vi "2B_Tech Serial Data Recording & DECADE 3.0.vi"() -> ()   [LabVIEW 2014]
uses:
  <vilib>/Instr/_visa.llb/VISA Set IO Buffer Mask.ctl
  <vilib>/Instr/_visa.llb/VISA Flush IO Buffer Mask.ctl
  <vilib>/Platform/TimedLoop/XDataNode/timing_clust.ctl
  <vilib>/Platform/TimedLoop/XDataNode/nitl_modes.ctl
  <vilib>/Platform/TimedLoop/XDataNode/wakeup.ctl
  C:/Program Files (x86)/National Instruments/LabVIEW 2014/examples/Data Communication/Network Streams/Simple Network Streams/support/Network Stream Command.ctl
  <vilib>/Utility/error.llb/whitespace.ctl
  <vilib>/Instr/_visa.llb/VISA Configure Serial Port (Instr).vi
  <vilib>/Utility/tcp.llb/UDP Multicast Write-Only Open.vi
  <vilib>/platform/TimedLoop/XDataNode/XDataNode.xnode
  <vilib>/Platform/TimedLoop/XDataNode/XDNodeRunTimeDep.lvlib
panel:
  out "SEPTIC TCP Error Out":errorcluster
  out "TCP packet\nSend to SEPTIC":bool
  in  "stop 2":bool
  out "FISH TCP Error Out":errorcluster
  out "TCP packet\nSend to FISH":bool
  in  "stop":bool
  out "Default file name":string
  out "error out":errorcluster
  out "Ambient/Cabin":bool
  out "Stop File Write":bool
  in  "timeout (10sec)":u32=3000
  in  "VISA resource name":refnum<visa-resource-name>="ASRL2::INSTR"
  out "Simulate 3 av":dbl
  out "Simulate\nConc":i32
  out "Simulate\nconc":bool
  out "3hr_alm_thresh":i32=80
  out "3hrAvg_Alarm":bool
  out "Inst_Alarm":bool
  out "Inst_alm_thresh":i32=220
  out "Time":string
  in  "Clear Display\nErrors":bool
  out "Read Error Counter\nfrom process loop":u32
  out "CABOZO UDP_ASCII_Out":string
  out "Ozo_array":string[](array[string])
  out "3hr_ozo_avg":dbl
  out "q_size":i32
  out "Data Output":string[](array[string])
  out "UDP packet\nSend status":bool
  out "TWBOZO UDP_ASCII_Out":string
  out "UDP_Out_Error":errorcluster
  out "UDP_Pack_num":u32
  out "Flight Number":string
  out "Number of times \nRead time out":u32
  out "Data Loop count":i32
  out "2B_Serial_error out":errorcluster
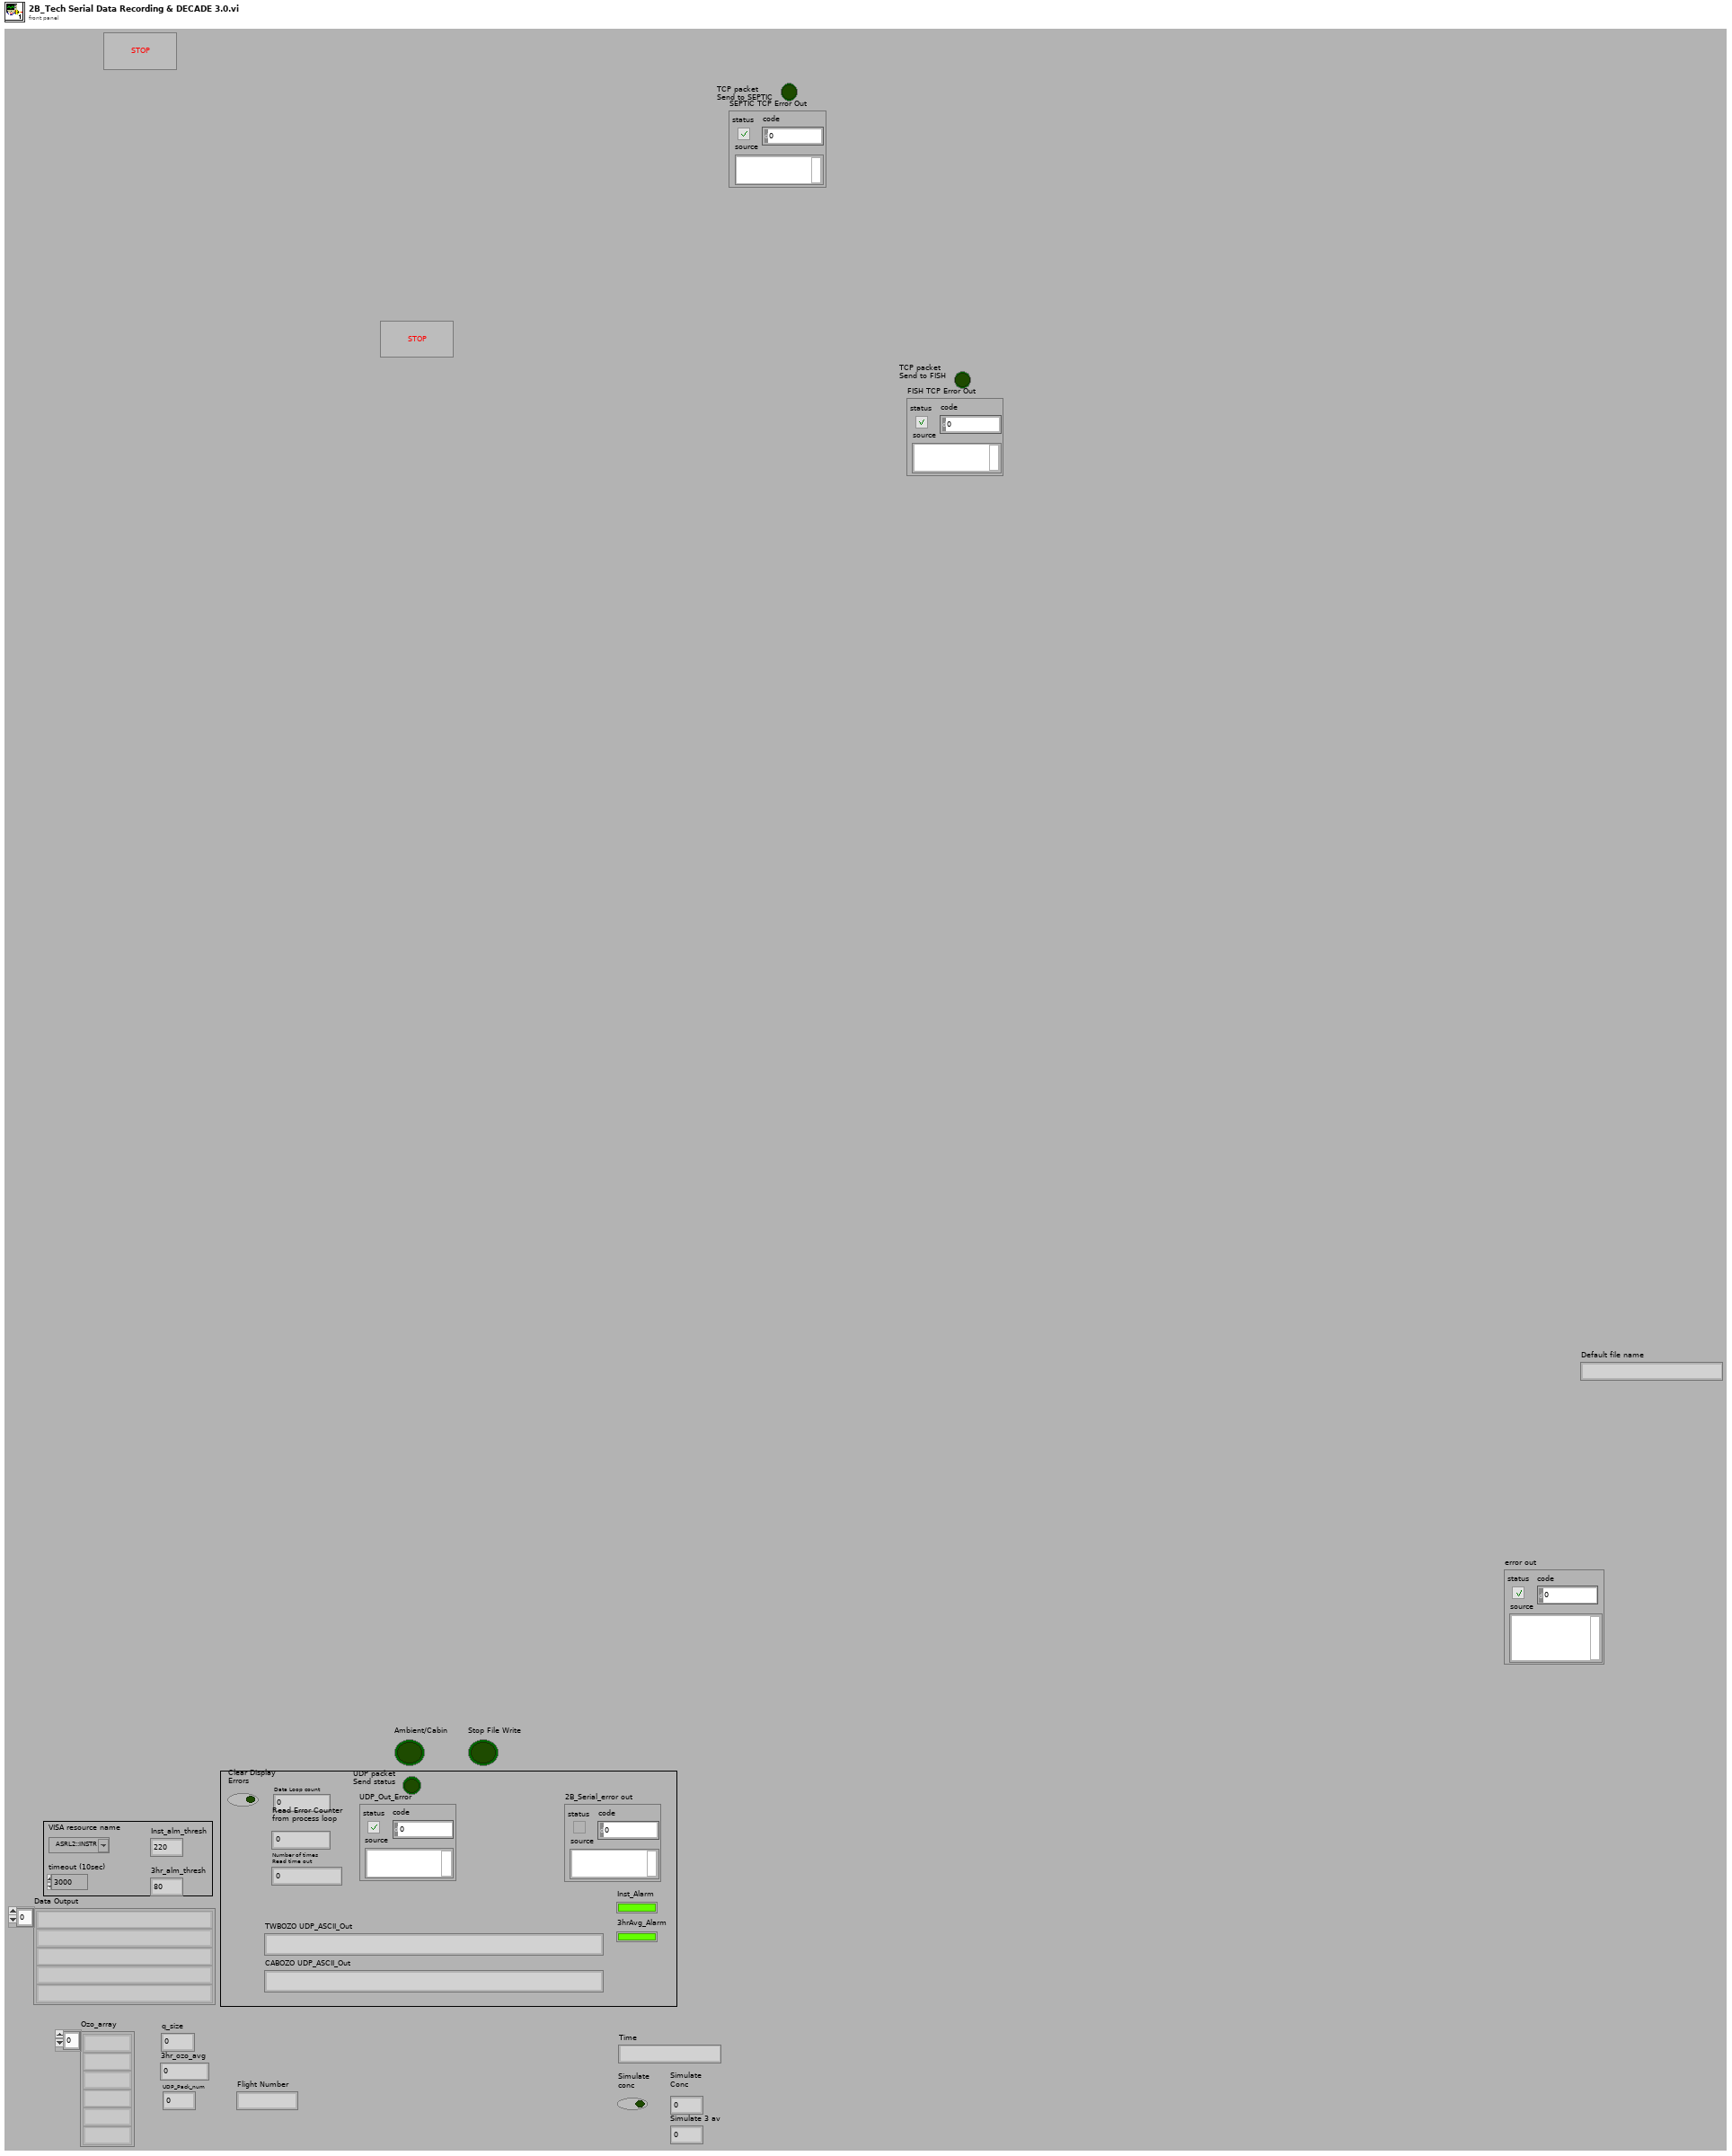
[diagram p1: front panel]
types:
  T1 = typedef "VISA Flush IO Buffer Mask.ctl" = u16
  T2 = typedef "VISA Set IO Buffer Mask.ctl" = u16
  T3 = typedef "XDNodeRunTimeDep.lvlib/timing_clust.ctl" = cluster{"Expected End [f-1]":u64, "Actual End [f-1]":u64, "Finished Late? [f-1]":bool, "Expected End [i-1]":u64, "Actual End [i-1]":u64, "Finished Late? [i-1]":bool, "Expected Start [i]":u64, "Actual Start [i]":u64, "Expected Start [f]":u64, "Actual Start [f]":u64, "Source Name":string, "Structure Name":string, "Period":i64, "Deadline":i64, "Offset":i64, "Start":i64, "Priority":i32, "Timeout":i32, "Mode":T4, "Wakeup Reason":T5, "Error":errorcluster, "Source Type":string, "Secondary Source Type":string, "Global End Time":u64, "Global Start Time":u64, "Frame Duration":u64, "Iteration Duration":u64, "Assigned CPU":i32, "I/O Scan Engine Mode":u32}
  T4 = typedef "XDNodeRunTimeDep.lvlib/nitl_modes.ctl" = enum32{"No Change", "Process missed periods, maintain original phase", "Discard missed periods, maintain original phase", "Process missed periods, ignore original phase", "Discard missed periods, ignore original phase"}
  T5 = typedef "XDNodeRunTimeDep.lvlib/wakeup.ctl" = enum32{"Normal", "Aborted", "Asynchronous wakeup", "Timing source error", "Timed loop error", "Timeout"}
  T6 = typedef "Network Stream Command.ctl" = cluster{"Message":string, "Message Data":variant}
  T7 = enum16{"open", "replace", "create", "open or create", "replace or create", "replace or create with confirmation"}
  T8 = typedef "whitespace.ctl" = u16
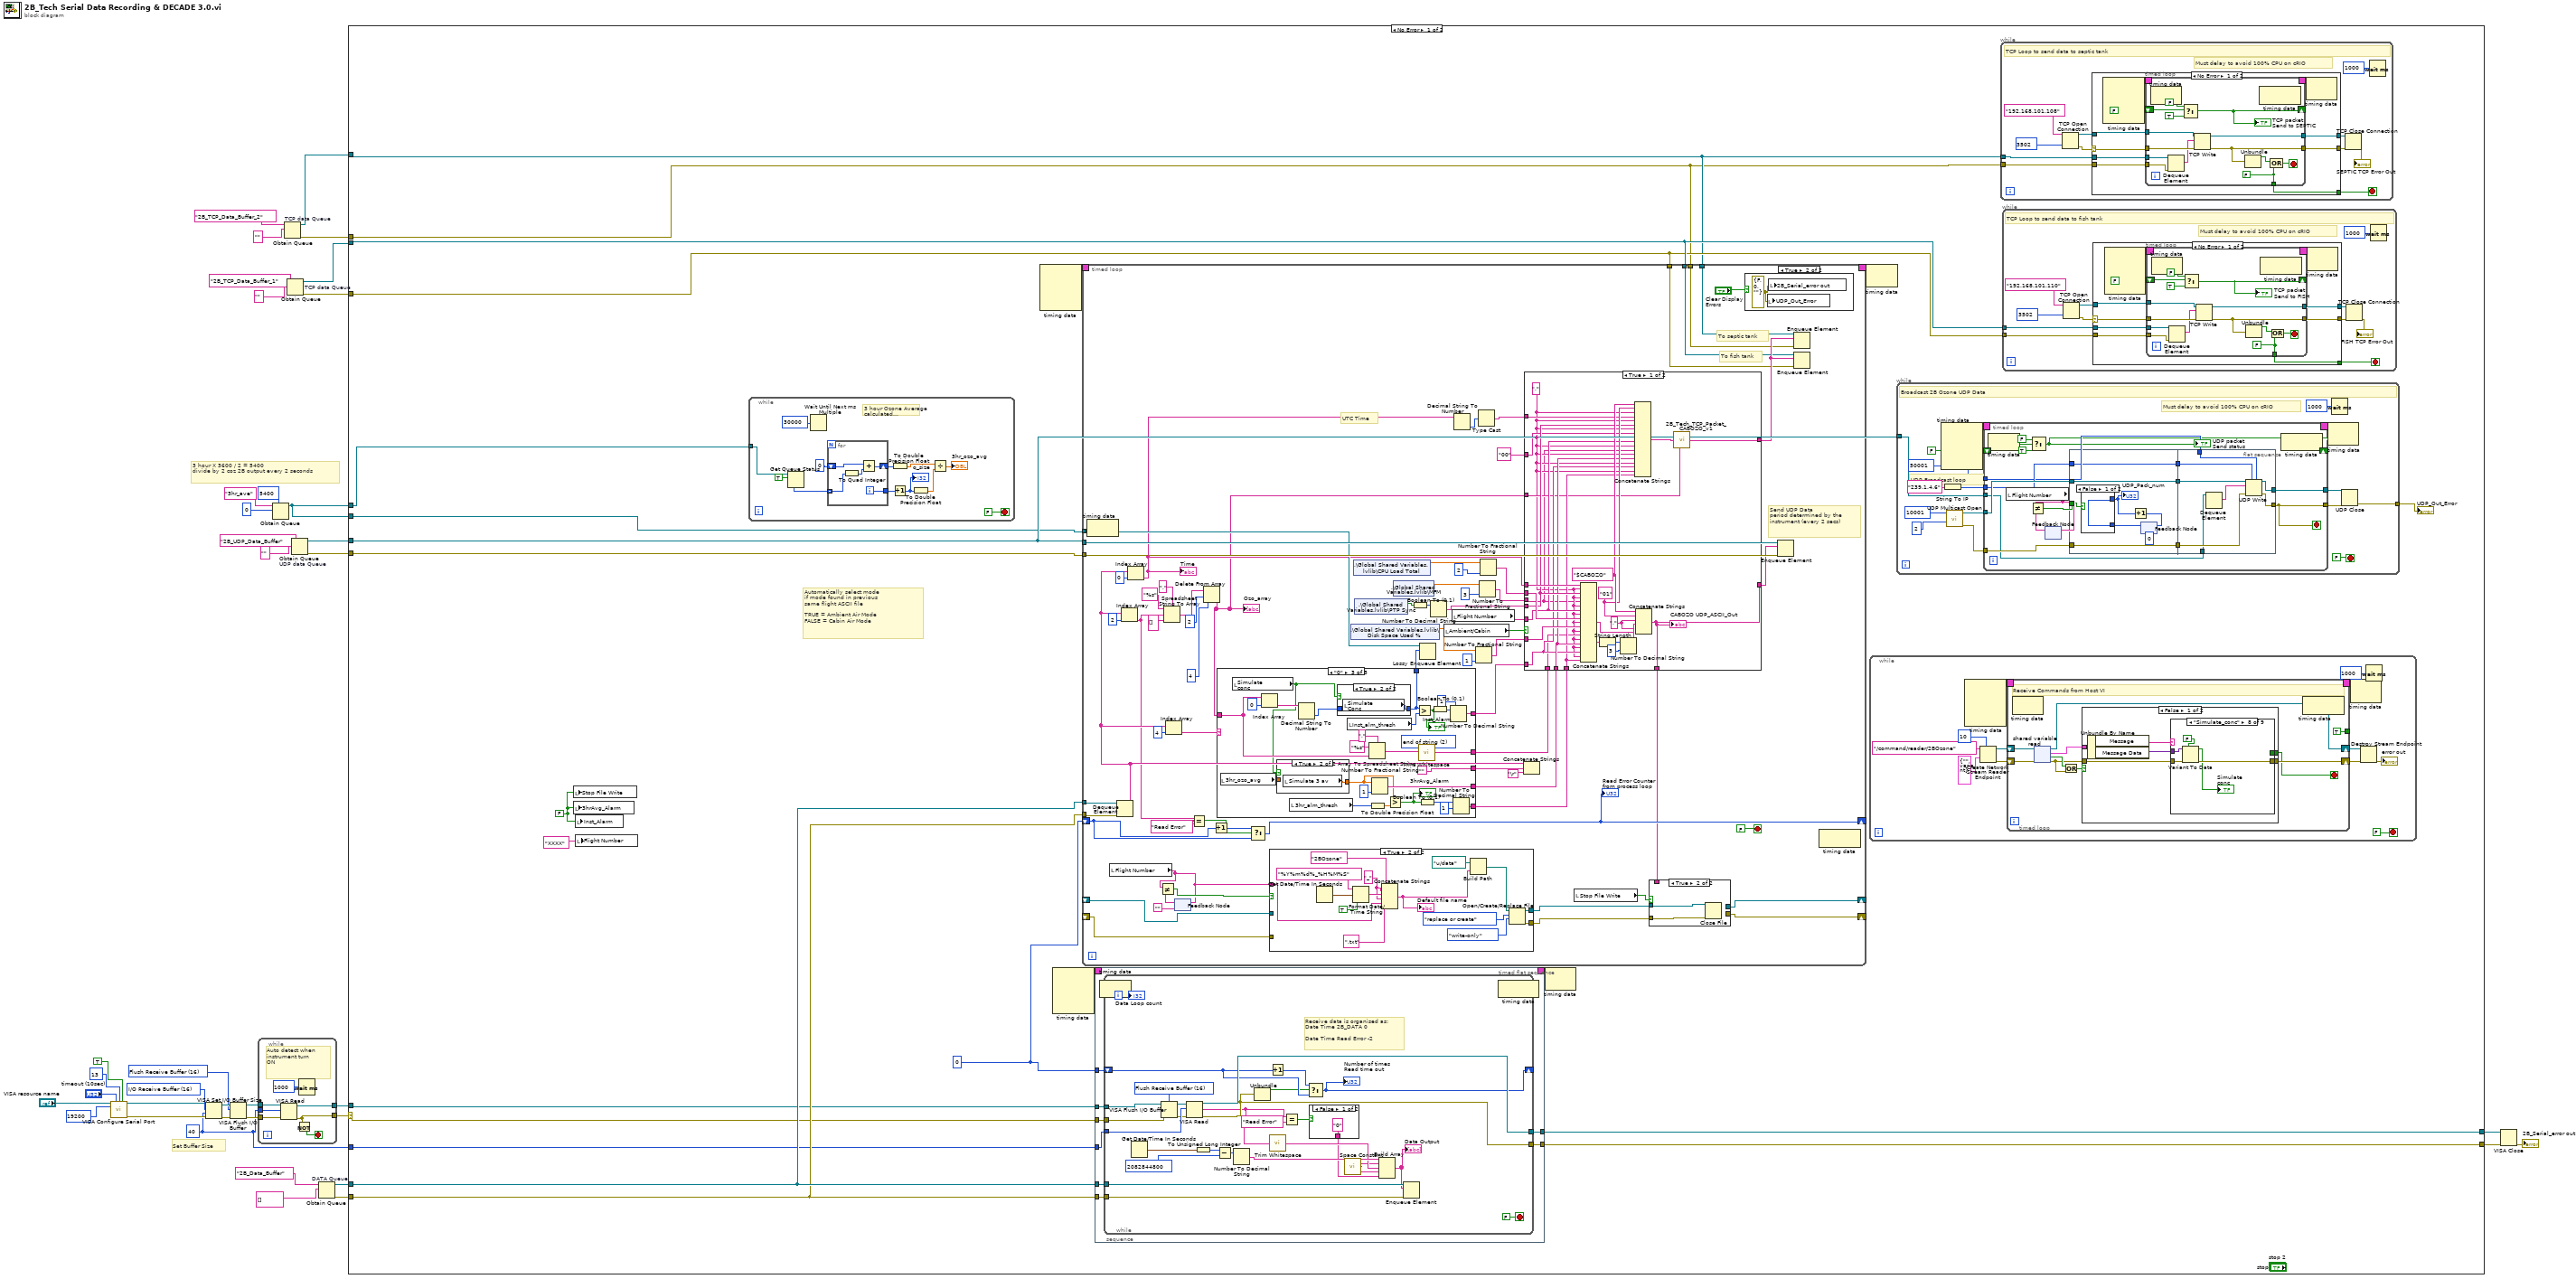
[diagram p0: block diagram]
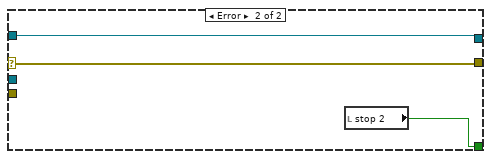
[diagram p2: hidden frame]
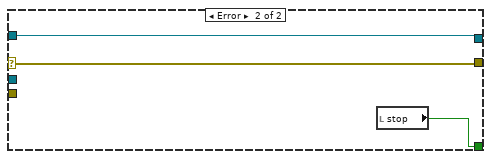
[diagram p3: hidden frame]
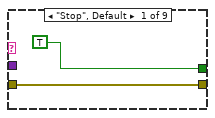
[diagram p4: hidden frame]
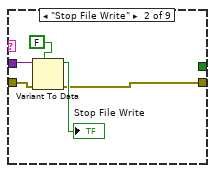
[diagram p5: hidden frame]
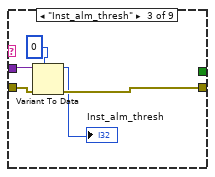
[diagram p6: hidden frame]
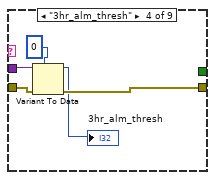
[diagram p7: hidden frame]
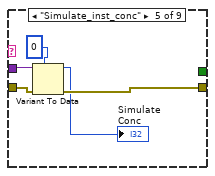
[diagram p8: hidden frame]
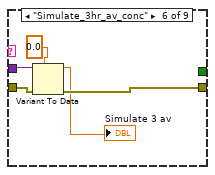
[diagram p9: hidden frame]
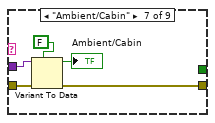
[diagram p10: hidden frame]
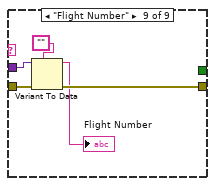
[diagram p11: hidden frame]
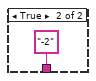
[diagram p13: hidden frame]
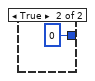
[diagram p14: hidden frame]
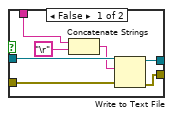
[diagram p15: hidden frame]
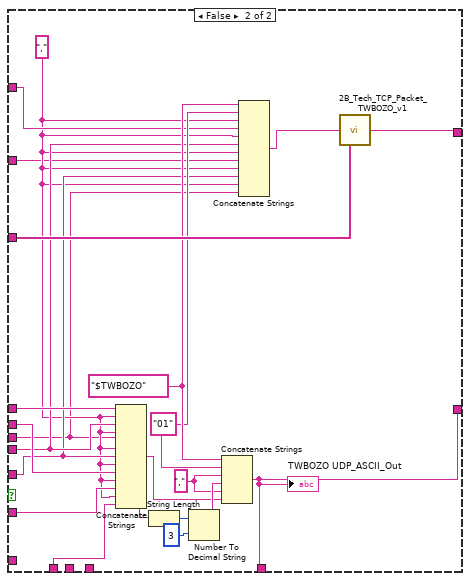
[diagram p18: hidden frame]
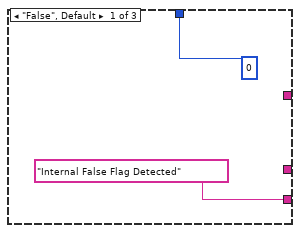
[diagram p19: hidden frame]
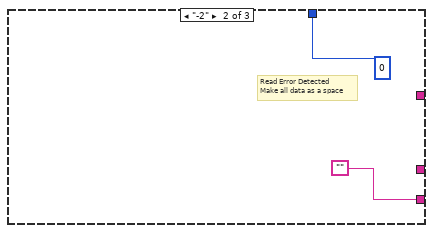
[diagram p20: hidden frame]
diagram:
  w9 = u32 40 ("size (4096)")
  w16 = T1 16 items=["Flush Receive Buffer"=16, "Write Transmit Buffer to Device"=32, "Flush Receive Buffer (No I/O)"=64, "Flush Transmit Buffer"=128] ("Mask")
  w17 = T2 16 items=["I/O Receive Buffer"=16, "I/O Transmit Buffer"=32, "I/O Receive and Transmit Buffer"=48] ("Mask")
  # "Set Buffer Size"
  # "3 hour X 3600 / 2 = 5400\ndivide by 2 coz 2B output every 2 seconds"
  n1 = call-poly "VISA Configure Serial Port"("VISA resource name"="VISA resource name", "timeout (10sec)"="timeout (10sec)", "termination char\n(0xA = '\\n' = LF)"=u8 13 ("termination char\n(0xA = '\\n' = LF)"), "Enable Termination\nChar (T)"=TRUE ("Enable Termination\nChar (T)"), "baud rate (9600)"=u32 19200) -> ("VISA resource name out"=w15:refnum<visa-resource-name>, "error out"=w14:errorcluster)  [unwired: 9 in]
  n2 = VISA Set I/O Buffer Size(VISA resource name=w15, mask (16)=w17, size (4096)=w9, error in (no error)=w14) -> (VISA resource name out=w18:refnum<visa-resource-name>, error out=w19:errorcluster)
  n3 = VISA Flush I/O Buffer(VISA resource name=w18, mask (16)=w16, error in (no error)=w19) -> (VISA resource name out=w13:refnum<visa-resource-name>, error out=w12:errorcluster)
  n4 = while {
    tunnel: w9 -> [w46]
    tunnel: w13 -> [w45]
    tunnel: w12 -> [w44]
    tunnel: [w42] -> w11
    tunnel: [w41] -> w10
    stop <- w43 stop-if-true
    # "Auto detect when\ninstrument turn\nON"
    n5 = VISA Read(VISA resource name=w45, byte count=w46, error in (no error)=w44) -> (VISA resource name out=w41:refnum<visa-resource-name>, error out=w42:errorcluster)  [unwired: 2 out]
    n6 = Not(x=w42) -> (.not. x?=w43:bool)
    n7 = Wait (ms)(milliseconds to wait=u32 1000) -> ()  [unwired: 1 out]
  }
  n8 = Obtain Queue(max queue size (-1, unlimited)=5400, name (unnamed)="3hr_ave", element data type=0 ("index")) -> (queue out=w25:refnum<queue>)  [unwired: 2 in, 2 out]
  n9 = Obtain Queue "TCP data Queue"(name (unnamed)="2B_TCP_Data_Buffer_2", element data type="") -> (queue out=w2:refnum<queue>, error out=w1:errorcluster)  [unwired: 3 in, 1 out]
  n10 = Obtain Queue "TCP data Queue"(name (unnamed)="2B_TCP_Data_Buffer_1", element data type="") -> (queue out=w4:refnum<queue>, error out=w3:errorcluster)  [unwired: 3 in, 1 out]
  n11 = Obtain Queue "UDP data Queue"(name (unnamed)="2B_UDP_Data_Buffer", element data type="") -> (queue out=w31:refnum<queue>, error out=w30:errorcluster)  [unwired: 3 in, 1 out]
  n12 = Obtain Queue "DATA Queue"(name (unnamed)="2B_Data_Buffer", element data type=string[] []) -> (queue out=w35:refnum<queue>, error out=w34:errorcluster)  [unwired: 3 in, 1 out]
  n13 = case shown="No Error" w11 {
    selector: w11 -> [w56 w531]
    tunnel: w10 -> [w57 w532]
    tunnel: [w69 w532] -> w38
    tunnel: [w61 w531] -> w39
    tunnel: w35 -> [w68 _]
    tunnel: w34 -> [w67 _]
    tunnel: w31 -> [w65 _]
    tunnel: w30 -> [w66 _]
    tunnel: w25 -> [w64 _]
    tunnel: w25 -> [w63 _]
    tunnel: w9 -> [w55 _]
    tunnel: w4 -> [w50 _]
    tunnel: w3 -> [w49 _]
    tunnel: w2 -> [w48 _]
    tunnel: w1 -> [w47 _]
    frame No Error {
      w52 = FALSE
      w62 = u32 0
      # "Automatically select mode\nif mode found in previous\nsame flight ASCII file\n\nTRUE = Ambient Air Mode\nFALSE = Cabin Air Mode"
      n14 = local write "Stop File Write"(w52) -> ()
      n15 = local write "3hrAvg_Alarm"(w52) -> ()
      n16 = local write "Inst_Alarm"(w52) -> ()
      n17 = local write "Flight Number"("XXXX" ("Flight Number")) -> ()
      n18 = while {
        tunnel: w64 -> [w284]
        stop <- FALSE stop-if-true
        # "3 hour Ozone Average calculated\nevery 30 seconds"
        n19 = Get Queue Status(queue=w284, return elements? (F)=TRUE) -> (elements=w281:i32[])  [unwired: 1 in, 7 out]
        n20 = Wait Until Next ms Multiple(millisecond multiple=u32 30000) -> ()  [unwired: 1 out]
        n21 = for {
          tunnel: [w296] -> w291
          shift-right: [w295] -> w289
          shift-left: i64 0 -> [w294]
          tunnel: w281 -> [w292] mode=indexing
          i -> [w296]
          n22 = To Quad Integer(1:w292) -> (0:w293:i64)
          n23 = Add(x=w294, y=w293) -> (x+y=w295:i64)
        }
        n24 = Increment(x=w291) -> (x+1=w285:i32)
        "q_size" <- w285
        n25 = To Double Precision Float(number=w289) -> (double precision float=w287:dbl)
        n26 = To Double Precision Float(number=w285) -> (double precision float=w288:dbl)
        n27 = Divide(x=w287, y=w288) -> (x/y=→"3hr_ozo_avg":dbl)
      }
      n28 = node-c288() -> (w60:T3)  [unwired: 4 in]
      n29 = node-c288() -> (w54:T3)  [unwired: 4 in]
      n30 = timed-loop {
        timing: w60 -> [_]
        timing-out: [_] -> w59
        tunnel: w68 -> [w419]
        tunnel: w67 -> [w418]
        tunnel: w65 -> [w417]
        tunnel: w66 -> [w416]
        tunnel: w63 -> [w390]
        shift-right: [w394] -> _
        shift-left: w62 -> [w395]
        shift-right: [w383] -> _
        shift-left: _ -> [w379]
        shift-right: [w377] -> _
        shift-left: _ -> [w378]
        tunnel: w50 -> [w356]
        tunnel: w49 -> [w355]
        tunnel: w48 -> [w354]
        tunnel: w47 -> [w353]
        stop <- FALSE stop-if-true
        # "UTC Time"
        # "To fish tank"
        # "To septic tank"
        # "Send UDP Data\nperiod determined by the\ninstrument (every 2 secs)"
        n31 = node-c288() -> ()  [unwired: 1 in, 1 out]
        n32 = local read "Flight Number"() -> (w375:string)
        n33 = Dequeue Element(queue=w419, error in (no error)=w418) -> (element=w403:string[])  [unwired: 1 in, 3 out]
        n34 = Index Array(array=w403, index=2) -> (element=w396:string)
        n35 = Index Array(array=w403, index=0) -> (element=w361:string)
        "Time" <- w361
        n36 = Spreadsheet String To Array(delimiter (Tab)=",", format string="%s", spreadsheet string=w396, array type (2D Dbl)=string[] [] ("Values Array")) -> (array=w408:string[])
        n37 = Index Array(array=w403, index=4) -> (element=w409:string)
        n38 = feedback #1("" ("Flight Number")) -> (w385:string)
        n39 = Not Equal?(x=w375, y=w385) -> (x != y?=w376:bool)
        n40 = feedback-in #1(w375) -> ()
        n41 = Equal?(x=w396, y="Read Error") -> (x = y?=w398:bool)
        n42 = Delete From Array(array=w408, length=2, index=4) -> (array with subset deleted=w358:string[])  [unwired: 1 out]
        "Ozo_array" <- w358
        n43 = Increment(x=w395) -> (x+1=w397:u32)
        n44 = case shown="\"0\"" w409 {
          tunnel: w358 -> [_ _ w515]
          tunnel: [_ _ w518] -> w404
          tunnel: [0 0 w503] -> w389
          tunnel: ["Internal False Flag Detected" "" ""] -> w402
          tunnel: [_ _ w512] -> w400
          tunnel: [_ _ w509] -> w392
          tunnel: [_ _ w505] -> w391
          frame "False", Default {
          }
          frame "-2" {
            # "Read Error Detected\nMake all data as a space"
          }
          frame "0" {
            w519 = T8 2 items=["both", "start of string", "end of string"] ("location (both)")
            n45 = local read "3hr_ozo_avg"() -> (w502:dbl)
            n46 = local read "Simulate\nconc"() -> (w498:bool)
            n47 = Index Array(array=w515, index=0) -> (element=w516:string)
            n48 = case shown="True" w498 {
              tunnel: [w523 w524] -> w501
              tunnel: w502 -> [w523 _]
              frame False {
              }
              frame True {
                n49 = local read "Simulate 3 av"() -> (w524:dbl)
              }
            }
            n50 = local read "3hr_alm_thresh"() -> (w499:i32)
            n51 = Decimal String To Number(string=w516) -> (number=w504:i32)  [unwired: 2 in, 1 out]
            n52 = case shown="True" w498 {
              tunnel: [w525 w526] -> w503
              tunnel: w504 -> [w525 _]
              frame False {
              }
              frame True {
                n53 = local read "Simulate\nConc"() -> (w526:i32)
              }
            }
            n54 = local read "Inst_alm_thresh"() -> (w500:i32)
            n55 = Array To Spreadsheet String(delimiter (Tab)=",", array=w515, 3:"%s" ("format string")) -> (spreadsheet string=w520:string)
            n56 = To Double Precision Float(number=w499) -> (double precision float=w506:dbl)
            n57 = Number To Fractional String(number=w501, precision (6)=i16 1) -> (F-format string=w512:string)  [unwired: 2 in]
            n58 = Greater?(x=w501, y=w506) -> (0:w507:bool)
            "3hrAvg_Alarm" <- w507
            n59 = Greater?(x=w503, y=w500) -> (0:w510:bool)
            "Inst_Alarm" <- w510
            n60 = call <vilib>:"Trim Whitespace.vi"("string"=w520, "location (both)"=w519) -> ("trimmed string"=w518:string)
            n61 = Boolean To (0,1)(Boolean=w507) -> (0, 1=w508:i16)
            n62 = Boolean To (0,1)(Boolean=w510) -> (0, 1=w511:i16)
            n63 = Number To Decimal String(number=w511, width (-)=i16 1) -> (decimal integer string=w509:string)
            n64 = Number To Decimal String(number=w508, width (-)=i16 1) -> (decimal integer string=w505:string)
          }
        }
        n65 = Select(t=w397, s=w398, f=w395) -> (s? t:f=w394:u32)
        "Read Error Counter\nfrom process loop" <- w394
        n66 = case shown="True" w376 {
          tunnel: [w430 w433] -> w381
          tunnel: [w429 w432] -> w380
          tunnel: w379 -> [w430 _]
          tunnel: w378 -> [w429 _]
          tunnel: w375 -> [_ w431]
          frame False {
          }
          frame True {
            w440 = "_" ("string")
            n67 = Get Date/Time In Seconds() -> (seconds since 1Jan1904=w441:timestamp)
            n68 = Format Date/Time String(time format string (%c)="%Y%m%d%_%H%M%S", seconds (now)=w441, UTC format=TRUE) -> (date/time string=w444:string)
            n69 = Concatenate Strings("2BOzone" ("string"), w440, w444, w440, w431, ".txt" ("string")) -> (w438:string)
            "Default file name" <- w438
            n70 = Build Path(base path=path "u:/data", name or relative path=w438) -> (appended path=w434:path)
            n71 = Open/Create/Replace File(file path (use dialog)=w434, operation (0:open)=T7."replace or create", access (0:read/write)=enum16{"read/write", "read-only", "write-only"}."write-only") -> (refnum out=w433:refnum<file>, error out=w432:errorcluster)  [unwired: 3 in, 1 out]
          }
        }
        n72 = shared-variable ".\\Global Shared Variables.lvlib\\Disk Space Used %"() -> (w363:dbl)  [unwired: 1 in, 1 out]
        n73 = shared-variable ".\\Global Shared Variables.lvlib\\CPU Load Total"() -> (w373:dbl)  [unwired: 1 in, 1 out]
        n74 = shared-variable ".\\Global Shared Variables.lvlib\\PTP Sync"() -> (w366:bool)  [unwired: 1 in, 1 out]
        n75 = shared-variable ".\\Global Shared Variables.lvlib\\MFM"() -> (w371:dbl)  [unwired: 1 in, 1 out]
        n76 = Boolean To (0,1)(Boolean=w366) -> (0, 1=w367:i16)
        n77 = Lossy Enqueue Element(queue=w390, element=w389) -> ()  [unwired: 1 in, 4 out]
        n78 = Number To Decimal String(number=w367) -> (decimal integer string=w365:string)  [unwired: 1 in]
        n79 = local read "Ambient/Cabin"() -> (w386:bool)
        n80 = local read "Flight Number"() -> (w387:string)
        n81 = Decimal String To Number(string=w361) -> (number=w360:i32)  [unwired: 2 in, 1 out]
        n82 = Number To Fractional String(number=w363, precision (6)=i16 1) -> (F-format string=w362:string)  [unwired: 2 in]
        n83 = Type Cast(x=w360) -> (*(type *) &x=w359:string)  [unwired: 1 in]
        n84 = Number To Fractional String(number=w371, precision (6)=i16 3) -> (F-format string=w368:string)  [unwired: 2 in]
        n85 = Number To Fractional String(number=w373, precision (6)=i16 2) -> (F-format string=w372:string)  [unwired: 2 in]
        n86 = Concatenate Strings(w403, w402, "\r") -> ()  [unwired: 1 out]
        n87 = case shown="True" w386 {
          tunnel: [w464 w485] -> w415
          tunnel: w361 -> [w465 w486]
          tunnel: w404 -> [w453 w482]
          tunnel: w372 -> [w463 w484]
          tunnel: w368 -> [w447 w471]
          tunnel: w387 -> [w457 w476]
          tunnel: w400 -> [w456 _]
          tunnel: w392 -> [w455 _]
          tunnel: w391 -> [w454 _]
          tunnel: [w464 w485] -> w374
          tunnel: w365 -> [w458 w477]
          tunnel: w362 -> [w462 w483]
          tunnel: w359 -> [w459 w478]
          tunnel: w358 -> [w450 w481]
          tunnel: [w451 w473] -> w357
          tunnel: "00" -> [w449 w472]
          frame True {
            w448 = ","
            w460 = "01"
            w467 = ","
            w461 = "$CABOZO"
            n88 = Concatenate Strings(w465, w448, w458, w448, w447, w448, w457, w448, w463, w448, w462, w448, w453, w448, w456, w448, w455, w448, w454) -> (w466:string)
            n89 = String Length(string=w466) -> (length=w470:i32)
            n90 = Number To Decimal String(number=w470, width (-)=i16 3) -> (decimal integer string=w468:string)
            n91 = Concatenate Strings(w461, w460, w448, w459, w448, w458, w448, w449, w448, w457, w448, w447, w448, w456, w448, w455, w448, w454) -> (w452:string)
            n92 = Concatenate Strings(w461, w460, w467, w468, w467, w466) -> (w464:string)
            "CABOZO UDP_ASCII_Out" <- w464
            n93 = call "2B_Tech_TCP_Packet_CABOZO_v1.vi"("TCP Packet In"=w452, "Data Array"=w450) -> ("TCP Binary Packet"=w451:string)  [unwired: 13 in]
          }
          frame False {
            w475 = ","
            w479 = "01"
            w488 = ","
            w480 = "$TWBOZO"
            n94 = Concatenate Strings(w486, w475, w477, w475, w471, w475, w476, w475, w484, w475, w483, w475, w482) -> (w487:string)
            n95 = String Length(string=w487) -> (length=w491:i32)
            n96 = Number To Decimal String(number=w491, width (-)=i16 3) -> (decimal integer string=w489:string)
            n97 = Concatenate Strings(w480, w479, w488, w489, w488, w487) -> (w485:string)
            "TWBOZO UDP_ASCII_Out" <- w485
            n98 = Concatenate Strings(w480, w479, w475, w478, w475, w477, w475, w472, w475, w476, w475, w471) -> (w474:string)
            n99 = call "2B_Tech_TCP_Packet_TWBOZO_v1.vi"("TCP Packet In"=w474, "Data Array"=w481) -> ("TCP Binary Packet"=w473:string)  [unwired: 13 in]
          }
        }
        n100 = local read "Stop File Write"() -> (w382:bool)
        n101 = case shown="True" w382 {
          tunnel: w381 -> [w426 w428]
          tunnel: w380 -> [w425 w427]
          tunnel: [w422 _] -> w383
          tunnel: [w421 _] -> w377
          tunnel: w374 -> [w420 _]
          frame False {
            n102 = Concatenate Strings(w420, "\r") -> (w423:string)
            n103 = Write to Text File(file (use dialog)=w426, text=w423, error in=w425) -> (refnum out=w422:refnum<file>, error out=w421:errorcluster)  [unwired: 2 out]
          }
          frame True {
            n104 = Close File(refnum=w428, error in=w427) -> ()  [unwired: 2 out]
          }
        }
        n105 = case shown="True" "Clear Display\nErrors" {
          frame False {
          }
          frame True {
            w446 = errorcluster {"status"=FALSE, "code"=0, "source"=""} ("UDP Error Out")
            n106 = local write "UDP_Out_Error"(w446) -> ()
            n107 = local write "2B_Serial_error out"(w446) -> ()
          }
        }
        n108 = Enqueue Element(queue=w417, element=w415, error in (no error)=w416) -> ()  [unwired: 1 in, 3 out]
        n109 = Enqueue Element(queue=w354, element=w357, error in (no error)=w353) -> ()  [unwired: 1 in, 3 out]
        n110 = Enqueue Element(queue=w356, element=w357, error in (no error)=w355) -> ()  [unwired: 1 in, 3 out]
        n111 = node-c288() -> ()  [unwired: 1 in, 1 out]
      }
      n112 = timed-sequence {
        timing: w54 -> [_]
        timing-out: [_] -> w53
        tunnel: [w237] -> w69
        tunnel: w68 -> [w236]
        tunnel: w67 -> [w235]
        tunnel: w62 -> [w234]
        tunnel: [w233] -> w61
        tunnel: w57 -> [w232]
        tunnel: w56 -> [w231]
        tunnel: w55 -> [w230]
        n113 = timed-flat-sequence {
          tunnel: [w245] -> w237
          tunnel: w236 -> [w244]
          tunnel: w235 -> [w243]
          tunnel: w234 -> [w242]
          tunnel: [w241] -> w233
          tunnel: w232 -> [w240]
          tunnel: w231 -> [w239]
          tunnel: w230 -> [w238]
          n114 = node-c288() -> ()  [unwired: 1 in, 1 out]
          n115 = while {
            tunnel: [w264] -> w241
            shift-right: [w270] -> _
            shift-left: w242 -> [w271]
            tunnel: [w273] -> w245
            tunnel: w240 -> [w269]
            tunnel: w239 -> [w268]
            tunnel: w244 -> [w267]
            tunnel: w243 -> [w266]
            tunnel: w238 -> [w265]
            i -> [w272]
            stop <- FALSE stop-if-true
            w249 = T1 16 items=["Flush Receive Buffer"=16, "Write Transmit Buffer to Device"=32, "Flush Receive Buffer (No I/O)"=64, "Flush Transmit Buffer"=128] ("Mask")
            # "Receive data is organised as:\nDate Time 2B_DATA 0\n\nDate Time Read Error -2"
            n116 = Get Date/Time In Seconds() -> (seconds since 1Jan1904=w259:timestamp)
            n117 = VISA Flush I/O Buffer(VISA resource name=w269, mask (16)=w249, error in (no error)=w268) -> (VISA resource name out=w250:refnum<visa-resource-name>, error out=w248:errorcluster)
            n118 = VISA Read(VISA resource name=w250, byte count=w265, error in (no error)=w248) -> (VISA resource name out=w273:refnum<visa-resource-name>, read buffer=w247:string, error out=w264:errorcluster)  [unwired: 1 out]
            n119 = To Unsigned Long Integer(number=w259) -> (unsigned 32bit integer=w261:u32)
            n120 = Subtract(x=w261, y=u32 2082844800) -> (x-y=w258:u32)
            n121 = Number To Decimal String(number=w258) -> (decimal integer string=w255:string)  [unwired: 1 in]
            n122 = Unbundle(w264) -> ("status"=w262:bool)  [unwired: 2 out]
            n123 = Increment(x=w271) -> (x+1=w263:u32)
            n124 = call <vilib>:"Trim Whitespace.vi"("string"=w247) -> ("trimmed string"=w254:string)  [unwired: 1 in]
            n125 = Equal?(x=w247, y="Read Error") -> (x = y?=w256:bool)
            n126 = Select(t=w263, s=w262, f=w271) -> (s? t:f=w270:u32)
            "Number of times \nRead time out" <- w270
            n127 = case shown="False" w256 {
              tunnel: ["0" "-2"] -> w252
              frame False {
              }
              frame True {
              }
            }
            n128 = call <vilib>:"Space Constant.vi"() -> ("String"=w253:string)
            n129 = Build Array(w255, w253, w254, w253, w252) -> (w251:string[])
            "Data Output" <- w251
            n130 = Enqueue Element(queue=w267, element=w251, error in (no error)=w266) -> ()  [unwired: 1 in, 3 out]
            "Data Loop count" <- w272
          }
          n131 = node-c288() -> ()  [unwired: 1 in, 1 out]
        }
      }
      n132 = node-c288(w53) -> ()  [unwired: 1 out]
      n133 = node-c288(w59) -> ()  [unwired: 1 out]
      n134 = while {
        stop <- FALSE stop-if-true
        n135 = node-c288() -> (w155:T3)  [unwired: 4 in]
        n136 = Create Network Stream Reader Endpoint(7:10 ("reader buffer size"), 9:T6 {"Message"="", "Message Data"=variant} ("Message Cluster"), 11:"/command/reader/2BOzone" ("reader url")) -> (0:w161:errorcluster, 3:w162:refnum<k21>)  [unwired: 4 in]
        n137 = timed-loop "Host->Target Command Reader" {
          shift-right: [w172] -> w159
          shift-left: w161 -> [w175]
          shift-right: [w173] -> w158
          shift-left: w162 -> [w174]
          tunnel: [TRUE] -> _
          timing: w155 -> [_]
          timing-out: [_] -> w154
          stop <- w166 stop-if-true
          # "Receive Commands from Host VI"
          n138 = node-c288() -> ()  [unwired: 1 in, 1 out]
          n139 = shared-variable-read(w174, w175) -> (w173:refnum<k21>, w168:errorcluster, w170:bool, w171:T6)  [unwired: 1 in]
          n140 = Or(x=w170, y=w168) -> (x .or. y?=w169:bool)
          n141 = case shown="False" w169 {
            selector: w169 -> [_ w226]
            tunnel: w168 -> [w183 w227]
            tunnel: [w182 w227] -> w172
            tunnel: w171 -> [w180 _]
            tunnel: [w181 w226] -> w166
            frame False {
              n142 = Unbundle By Name(w180) -> ("Message"=w179:string, "Message Data"=w178:variant)
              n143 = case shown="\"Simulate_conc\"" w179 {
                tunnel: w183 -> [w185 w190 w195 w200 w205 w210 w215 w220 w225]
                tunnel: [w185 w186 w193 w198 w203 w208 w214 w219 w224] -> w182
                tunnel: w178 -> [_ w189 w194 w199 w204 w209 w213 w218 w223]
                tunnel: [TRUE _ _ _ _ _ _ _ _] -> w181
                frame "Stop", Default {
                }
                frame "Stop File Write" {
                  n144 = Variant To Data(error in=w190, type=FALSE, Variant=w189) -> (data=→"Stop File Write":bool, error out=w186:errorcluster)
                }
                frame "Inst_alm_thresh" {
                  n145 = Variant To Data(error in=w195, type=0, Variant=w194) -> (data=→"Inst_alm_thresh":i32, error out=w193:errorcluster)
                }
                frame "3hr_alm_thresh" {
                  n146 = Variant To Data(error in=w200, type=0, Variant=w199) -> (data=→"3hr_alm_thresh":i32, error out=w198:errorcluster)
                }
                frame "Simulate_inst_conc" {
                  n147 = Variant To Data(error in=w205, type=0, Variant=w204) -> (data=→"Simulate\nConc":i32, error out=w203:errorcluster)
                }
                frame "Simulate_3hr_av_conc" {
                  n148 = Variant To Data(error in=w210, type=0.0, Variant=w209) -> (data=→"Simulate 3 av":dbl, error out=w208:errorcluster)
                }
                frame "Ambient/Cabin" {
                  n149 = Variant To Data(error in=w215, type=FALSE, Variant=w213) -> (data=→"Ambient/Cabin":bool, error out=w214:errorcluster)
                }
                frame "Simulate_conc" {
                  n150 = Variant To Data(error in=w220, type=FALSE, Variant=w218) -> (data=→"Simulate\nconc":bool, error out=w219:errorcluster)
                }
                frame "Flight Number" {
                  n151 = Variant To Data(error in=w225, type="", Variant=w223) -> (data=→"Flight Number":string, error out=w224:errorcluster)
                }
              }
            }
            frame True {
            }
          }
          n152 = node-c288() -> ()  [unwired: 1 in, 1 out]
        }
        n153 = node-c288(w154) -> ()  [unwired: 1 out]
        n154 = Destroy Stream Endpoint(8:w159, 11:w158) -> (0:→"error out":errorcluster)
        n155 = Wait (ms)(milliseconds to wait=u32 1000) -> ()  [unwired: 1 out]
      }
      n156 = while {
        tunnel: w65 -> [w300]
        tunnel: [w299] -> w58
        stop <- FALSE stop-if-true
        # "Must delay to avoid 100% CPU on cRIO"
        # "UDP Broadcast loop"
        # "Broadcast 2B Ozone UDP Data"
        n157 = node-c288() -> (w302:T3)  [unwired: 4 in]
        n158 = String To IP(1:"239.1.4.6" ("name")) -> (0:w304:u32)
        n159 = call-poly <vilib>:"UDP Multicast Open.vi"("time-to-live (1)"=u16 2, "port"=u16 10001) -> ("error out"=w311:errorcluster, "connection ID"=w312:refnum<k16>)  [unwired: 8 in]
        n160 = timed-loop {
          tunnel: w312 -> [w329]
          tunnel: w311 -> [w328]
          tunnel: [w317] -> w307
          shift-right: [w314] -> _
          shift-left: FALSE -> [w322]
          tunnel: [w313] -> w306
          tunnel: w304 -> [w319]
          tunnel: u16 50001 ("port or service name") -> [w318]
          timing: w302 -> [_]
          timing-out: [_] -> w301
          tunnel: w300 -> [w315]
          stop <- w313 stop-if-true
          n161 = node-c288() -> ()  [unwired: 1 in, 1 out]
          n162 = local read "Flight Number"() -> (w316:string)
          n163 = Select(t=FALSE, s=w322, f=TRUE) -> (s? t:f=w314:bool)
          "UDP packet\nSend status" <- w314
          n164 = feedback-in #2(w316) -> ()
          n165 = feedback #2() -> (w324:string)  [unwired: 1 in]
          n166 = Not Equal?(x=w316, y=w324) -> (x != y?=w323:bool)
          n167 = flat-sequence {
            tunnel: w319 -> [w337]
            tunnel: w328 -> [w338]
            tunnel: w329 -> [w339]
            tunnel: [w339] -> w327
            tunnel: [w338] -> w326
            tunnel: [w337] -> w325
            tunnel: w323 -> [w336]
            tunnel: w318 -> [w349]
            tunnel: w327 -> [w348]
            tunnel: w326 -> [w347]
            tunnel: w325 -> [w346]
            tunnel: [w345] -> w317
            tunnel: [w344] -> w313
            tunnel: w315 -> [w342]
            frame #0 {
              n168 = feedback #3(u32 0) -> (w333:u32)
              n169 = case shown="False" w336 {
                tunnel: w333 -> [w340 _]
                tunnel: [w340 u32 0] -> w332
                frame False {
                }
                frame True {
                }
              }
              "UDP_Pack_num" <- w332
              n170 = Increment(x=w332) -> (x+1=w334:u32)
              n171 = feedback-in #3(w334) -> ()
            }
            frame #1 {
              n172 = Dequeue Element(queue=w342) -> (element=w343:string)  [unwired: 2 in, 3 out]
              n173 = UDP Write(address=w346, port or service name=w349, connection ID=w348, data in=w343, 8:w347) -> (error out=w344:errorcluster, 3:w345:refnum<k16>)  [unwired: 1 in]
            }
          }
          n174 = node-c288() -> ()  [unwired: 1 in, 1 out]
        }
        n175 = node-c288(w301) -> ()  [unwired: 1 out]
        n176 = Wait (ms)(milliseconds to wait=u32 1000) -> ()  [unwired: 1 out]
        n177 = UDP Close(connection ID=w307, 8:w306) -> (error out=w299:errorcluster)  [unwired: 1 out]
      }
      "UDP_Out_Error" <- w58
      n178 = while {
        tunnel: w47 -> [w72]
        tunnel: w48 -> [w71]
        stop <- w75 stop-if-true
        # "Must delay to avoid 100% CPU on cRIO"
        # "TCP Loop to send data to septic tank"
        n179 = TCP Open Connection(address="192.168.101.108", remote port or service name=u16 3502) -> (connection ID=w78:refnum<k5>, error out=w73:errorcluster)  [unwired: 3 in]
        n180 = case shown="No Error" w73 {
          selector: w73 -> [w83 w110]
          tunnel: w78 -> [w88 w111]
          tunnel: [w87 w111] -> w77
          tunnel: [w86 w110] -> w76
          tunnel: [w85 w109] -> w75
          tunnel: w71 -> [w82 _]
          tunnel: w72 -> [w81 _]
          frame No Error {
            n181 = node-c288() -> (w90:T3)  [unwired: 4 in]
            n182 = timed-loop {
              tunnel: w88 -> [w104]
              tunnel: w83 -> [w103]
              tunnel: [w102] -> w87
              tunnel: [w101] -> w86
              tunnel: [w91] -> w85
              shift-right: [w95] -> _
              shift-left: FALSE -> [w98]
              timing: w90 -> [_]
              timing-out: [_] -> w89
              tunnel: w82 -> [w94]
              tunnel: w81 -> [w93]
              stop <- w99 stop-if-true
              w91 = FALSE
              n183 = node-c288() -> ()  [unwired: 1 in, 1 out]
              n184 = Dequeue Element(queue=w94, error in (no error)=w93) -> (element=w92:string)  [unwired: 1 in, 3 out]
              n185 = Select(t=FALSE, s=w98, f=TRUE) -> (s? t:f=w95:bool)
              "TCP packet\nSend to SEPTIC" <- w95
              n186 = TCP Write(connection ID=w104, data in=w92, error in (no error)=w103) -> (connection ID out=w102:refnum<k5>, error out=w101:errorcluster)  [unwired: 1 in, 1 out]
              n187 = Unbundle(w101) -> ("status"=w100:bool)  [unwired: 2 out]
              n188 = node-c288() -> ()  [unwired: 1 in, 1 out]
              n189 = Compound Arithmetic op=OR(w100, w91) -> (w99:bool)
            }
            n190 = node-c288(w89) -> ()  [unwired: 1 out]
          }
          frame Error {
            n191 = local read "stop 2"() -> (w109:bool)
          }
        }
        n192 = TCP Close Connection(connection ID=w77, error in (no error)=w76) -> (error out=→"SEPTIC TCP Error Out":errorcluster)  [unwired: 1 in, 1 out]
        n193 = Wait (ms)(milliseconds to wait=u32 1000) -> ()  [unwired: 1 out]
      }
      n194 = while {
        tunnel: w50 -> [w114]
        tunnel: w49 -> [w113]
        stop <- w117 stop-if-true
        # "Must delay to avoid 100% CPU on cRIO"
        # "TCP Loop to send data to fish tank"
        n195 = TCP Open Connection(address="192.168.101.110", remote port or service name=u16 3502) -> (connection ID=w120:refnum<k5>, error out=w115:errorcluster)  [unwired: 3 in]
        n196 = case shown="No Error" w115 {
          selector: w115 -> [w125 w152]
          tunnel: w120 -> [w130 w153]
          tunnel: [w129 w153] -> w119
          tunnel: [w128 w152] -> w118
          tunnel: [w127 w151] -> w117
          tunnel: w114 -> [w124 _]
          tunnel: w113 -> [w123 _]
          frame No Error {
            n197 = node-c288() -> (w132:T3)  [unwired: 4 in]
            n198 = timed-loop {
              tunnel: w130 -> [w146]
              tunnel: w125 -> [w145]
              tunnel: [w144] -> w129
              tunnel: [w143] -> w128
              tunnel: [w140] -> w127
              shift-right: [w136] -> _
              shift-left: FALSE -> [w139]
              timing: w132 -> [_]
              timing-out: [_] -> w131
              tunnel: w124 -> [w135]
              tunnel: w123 -> [w134]
              stop <- w141 stop-if-true
              w140 = FALSE
              n199 = node-c288() -> ()  [unwired: 1 in, 1 out]
              n200 = Dequeue Element(queue=w135, error in (no error)=w134) -> (element=w133:string)  [unwired: 1 in, 3 out]
              n201 = Select(t=FALSE, s=w139, f=TRUE) -> (s? t:f=w136:bool)
              "TCP packet\nSend to FISH" <- w136
              n202 = TCP Write(connection ID=w146, data in=w133, error in (no error)=w145) -> (connection ID out=w144:refnum<k5>, error out=w143:errorcluster)  [unwired: 1 in, 1 out]
              n203 = Unbundle(w143) -> ("status"=w142:bool)  [unwired: 2 out]
              n204 = node-c288() -> ()  [unwired: 1 in, 1 out]
              n205 = Compound Arithmetic op=OR(w142, w140) -> (w141:bool)
            }
            n206 = node-c288(w131) -> ()  [unwired: 1 out]
          }
          frame Error {
            n207 = local read "stop"() -> (w151:bool)
          }
        }
        n208 = TCP Close Connection(connection ID=w119, error in (no error)=w118) -> (error out=→"FISH TCP Error Out":errorcluster)  [unwired: 1 in, 1 out]
        n209 = Wait (ms)(milliseconds to wait=u32 1000) -> ()  [unwired: 1 out]
      }
    }
    frame Error {
    }
  }
  n210 = VISA Close(VISA resource name=w38, error in (no error)=w39) -> (error out=→"2B_Serial_error out":errorcluster)
